vi "ECS - TDK_HVPS_Control.vi"(4 "VISA In":refnum<visa-resource-name>="COM1") -> ()   [LabVIEW 2015, in "ECS-RT.lvlib"]
uses:
  ECS-RT.lvlib
panel:
  out "error out":errorcluster {"code" format="%.0x"}
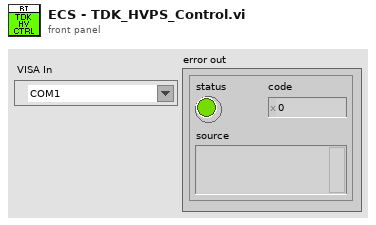
[diagram p1: front panel]
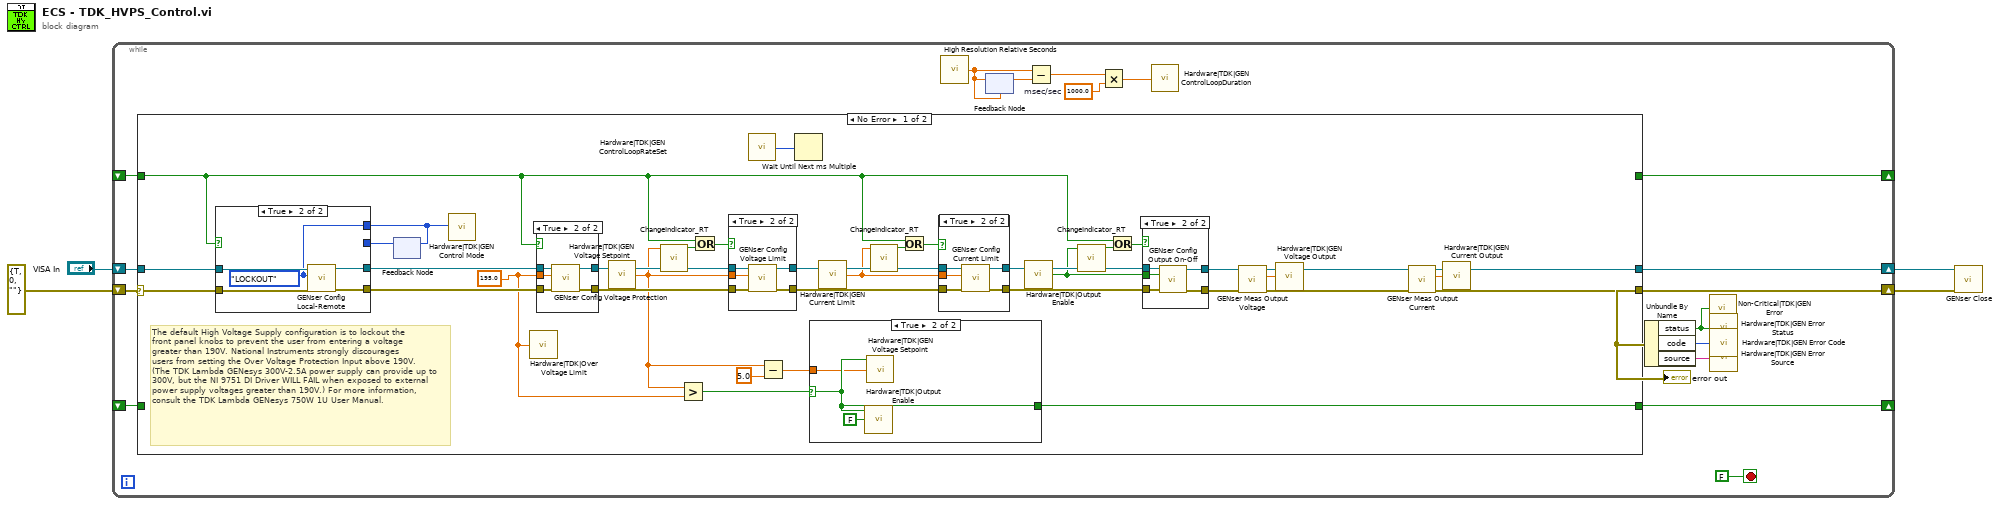
[diagram p0: block diagram]
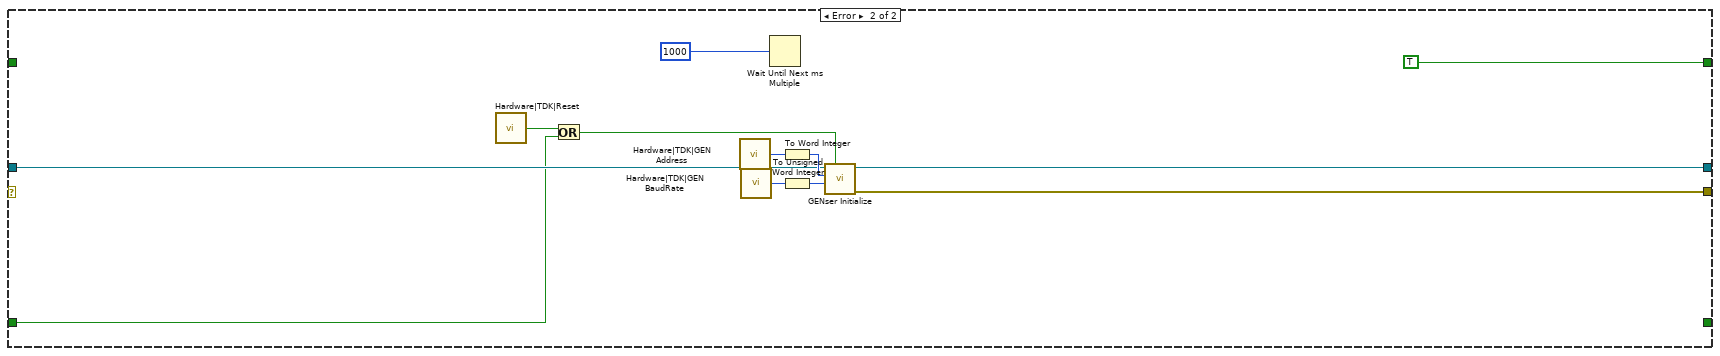
[diagram p8: hidden frame]
diagram:
  n1 = while {
    shift-right: [w14] -> w2
    shift-left: "VISA In" -> [w16]
    shift-right: [w6] -> w1
    shift-left: errorcluster {"status"=TRUE, "code"=0, "source"=""} ("error constant") -> [w15]
    shift-right: [w13] -> _
    shift-left: _ -> [w12]
    shift-right: [w11] -> _
    shift-left: _ -> [w10]
    stop <- FALSE stop-if-true
    w21 = 1000.0  # msec/sec
    n2 = case shown="No Error" w15 {
      selector: w15 -> [w39 _]
      tunnel: [w57 w100] -> w14
      tunnel: [w41 w101] -> w6
      tunnel: w16 -> [w56 w103]
      tunnel: [_ TRUE] -> w13
      tunnel: w12 -> [w25 _]
      tunnel: [w30 _] -> w11
      tunnel: w10 -> [_ w97]
      frame No Error {
        w24 = sgl 195.0 ("Value")
        # "The default High Voltage Supply configuration is to lockout the \nfront panel knobs to prevent the user from entering a voltage \ngreater than 190V. National Instruments strongly discourages \nusers from setting the Over Voltage Protection Input above 190V. (The TDK Lambda GENesys 300V-2.5A power supply can provide up to 300V, but the NI 9751 DI Driver WILL FAIL when exposed to external power supply voltages greater than 190V.) For more information, consult the TDK Lambda GENesys 750W 1U User Manual."
        n3 = feedback #1() -> (w22:enum16{"LOCAL", "REMOTE", "LOCKOUT"})  [unwired: 1 in]
        n4 = case shown="True" w25 {
          tunnel: w56 -> [w60 w65]
          tunnel: [w59 w64] -> w45
          tunnel: [w60 w63] -> w44
          tunnel: w39 -> [w59 w62]
          tunnel: [w58 w61] -> w23
          tunnel: w22 -> [w58 _]
          frame False {
          }
          frame True {
            w61 = enum16{"LOCAL", "REMOTE", "LOCKOUT"}."LOCKOUT" ("Mode")
            n5 = call <instrlib>:"GENser Config Local-Remote.vi"("error"=w62, "Mode"=w61, "VISA"=w65) -> ("error out"=w64:errorcluster, "VISA out"=w63:refnum<visa-resource-name>)  [unwired: 7 in]
          }
        }
        n6 = feedback-in #1(w23) -> ()
        n7 = call "Hardware|TDK|GEN Control Mode"("Value"=w23) -> ()
        n8 = call "Hardware|TDK|Over Voltage Limit"("Value"=w24) -> ()
        n9 = case shown="True" w25 {
          tunnel: w45 -> [w90 w96]
          tunnel: w44 -> [w91 w95]
          tunnel: [w91 w94] -> w43
          tunnel: [w90 w93] -> w42
          tunnel: w24 -> [_ w92]
          frame False {
          }
          frame True {
            n10 = call <instrlib>:"GENser Config Voltage Protection.vi"("error"=w96, "OVP Level"=w92, "VISA"=w95) -> ("error out"=w93:errorcluster, "VISA out"=w94:refnum<visa-resource-name>)  [unwired: 7 in]
          }
        }
        n11 = call "Hardware|TDK|GEN Voltage Setpoint"() -> ("Value"=w27:sgl)
        n12 = call "ChangeIndicator_RT.vi"("Input"=w27) -> ("Change"=w38:bool)  [unwired: 9 in]
        n13 = Greater?(x=w27, y=w24) -> (0:w26:bool)
        n14 = Or(x=w25, y=w38) -> (x .or. y?=w37:bool)
        n15 = case shown="True" w37 {
          tunnel: [w83 w89] -> w51
          tunnel: [w84 w88] -> w50
          tunnel: w27 -> [_ w87]
          tunnel: w43 -> [w84 w86]
          tunnel: w42 -> [w83 w85]
          frame False {
          }
          frame True {
            n16 = call <instrlib>:"GENser Config Voltage Limit.vi"("error"=w85, "Volt Limit"=w87, "VISA"=w86) -> ("error out"=w89:errorcluster, "VISA out"=w88:refnum<visa-resource-name>)  [unwired: 7 in]
          }
        }
        n17 = call "Hardware|TDK|GEN ControlLoopRateSet"() -> ("Value"=w40:u32)
        n18 = Subtract(x=w27, y=sgl 5.0) -> (x-y=w28:sgl)
        n19 = Wait Until Next ms Multiple(millisecond multiple=w40) -> ()  [unwired: 1 out]
        n20 = case shown="True" w26 {
          selector: w26 -> [_ w68]
          tunnel: [_ w68] -> w30
          tunnel: w28 -> [_ w66]
          frame False {
          }
          frame True {
            n21 = call "Hardware|TDK|Output Enable"("Value"=FALSE, "Adapt"=w68) -> ()  [unwired: 1 in]
            n22 = call "Hardware|TDK|GEN Voltage Setpoint"("Value"=w66, "Adapt"=w68) -> ()  [unwired: 1 in]
          }
        }
        n23 = call "Hardware|TDK|GEN Current Limit"() -> ("Value"=w34:sgl)
        n24 = call "ChangeIndicator_RT.vi"("Input"=w34) -> ("Change"=w35:bool)  [unwired: 9 in]
        n25 = Or(x=w25, y=w35) -> (x .or. y?=w36:bool)
        n26 = case shown="True" w36 {
          tunnel: [w76 w82] -> w53
          tunnel: [w77 w81] -> w52
          tunnel: w51 -> [w76 w80]
          tunnel: w50 -> [w77 w79]
          tunnel: w34 -> [_ w78]
          frame False {
          }
          frame True {
            n27 = call <instrlib>:"GENser Config Current Limit.vi"("error"=w80, "Current Limit"=w78, "VISA"=w79) -> ("error out"=w82:errorcluster, "VISA out"=w81:refnum<visa-resource-name>)  [unwired: 7 in]
          }
        }
        n28 = call "Hardware|TDK|Output Enable"() -> ("Value"=w31:bool)
        n29 = call "ChangeIndicator_RT.vi"("Input"=w31) -> ("Change"=w32:bool)  [unwired: 9 in]
        n30 = Or(x=w25, y=w32) -> (x .or. y?=w33:bool)
        n31 = case shown="True" w33 {
          tunnel: w53 -> [w69 w75]
          tunnel: w52 -> [w70 w74]
          tunnel: [w70 w73] -> w49
          tunnel: [w69 w72] -> w48
          tunnel: w31 -> [_ w71]
          frame False {
          }
          frame True {
            n32 = call <instrlib>:"GENser Config Output On-Off.vi"("error"=w75, "Output ON"=w71, "VISA"=w74) -> ("error out"=w72:errorcluster, "VISA out"=w73:refnum<visa-resource-name>)  [unwired: 7 in]
          }
        }
        n33 = call <instrlib>:"GENser Meas Output Voltage.vi"("error"=w48, "VISA"=w49) -> ("error out"=w55:errorcluster, "Output Voltage"=w47:dbl, "VISA out"=w54:refnum<visa-resource-name>)  [unwired: 7 in]
        n34 = call "Hardware|TDK|GEN Voltage Output"("Value"=w47) -> ()
        n35 = call <instrlib>:"GENser Meas Output Current.vi"("error"=w55, "VISA"=w54) -> ("error out"=w41:errorcluster, "Output Current"=w46:dbl, "VISA out"=w57:refnum<visa-resource-name>)  [unwired: 7 in]
        n36 = call "Hardware|TDK|GEN Current Output"("Value"=w46) -> ()
      }
      frame Error {
        n37 = call "Hardware|TDK|Reset"() -> ("Value"=w108:bool)
        n38 = Or(x=w108, y=w97) -> (x .or. y?=w98:bool)
        n39 = call "Hardware|TDK|GEN Address"() -> ("Value"=w105:i32)
        n40 = call "Hardware|TDK|GEN BaudRate"() -> ("Value"=w104:u32)
        n41 = Wait Until Next ms Multiple(millisecond multiple=u32 1000) -> ()  [unwired: 1 out]
        n42 = To Word Integer(number=w105) -> (16bit integer=w106:i16)
        n43 = To Unsigned Word Integer(number=w104) -> (unsigned 16bit integer=w107:u16)
        n44 = call <instrlib>:"GENser Initialize.vi"("Reset (T)"=w98, "BAUD"=w107, "GEN Addr"=w106, "VISA name"=w103) -> ("error out"=w101:errorcluster, "VISA out"=w100:refnum<visa-resource-name>)  [unwired: 6 in]
      }
    }
    "error out" <- w6
    n45 = call <vilib>:"High Resolution Relative Seconds.vi"() -> ("relative seconds"=w19:dbl)
    n46 = feedback #2(w19) -> (w18:dbl)
    n47 = feedback-in #2(w19) -> ()
    n48 = Subtract(x=w19, y=w18) -> (x-y=w20:dbl)
    n49 = Multiply(x=w20, y=w21) -> (x*y=w17:dbl)
    n50 = call "Hardware|TDK|GEN ControlLoopDuration"("Value"=w17) -> ()
    n51 = Unbundle By Name(w6) -> ("status"=w7:bool, "code"=w8:i32, "source"=w9:string)
    n52 = call "Non-Critical|TDK|GEN Error"("Fault"=w7) -> ()  [unwired: 2 in]
    n53 = call "Hardware|TDK|GEN Error Status"("Value"=w7) -> ()
    n54 = call "Hardware|TDK|GEN Error Code"("Value"=w8) -> ()
    n55 = call "Hardware|TDK|GEN Error Source"("Value"=w9) -> ()
  }
  n56 = call <instrlib>:"GENser Close.vi"("error"=w1, "VISA name"=w2) -> ()  [unwired: 9 in, 1 out]
